vi "CONTROL TARGETING.vi"(8 "error in (no error)":errorcluster, 11 "control\ncluster":T1) -> (0 "error out":errorcluster, 3 "control\ncluster out":T1)   [LabVIEW 2023]
uses:
  ctrl defs/ctrl controllers.ctl
  Global odometry.vi
panel:
  in  "notes":string="ffsdfsdfsdf sdf sfsdf sdfsd sfds f sf sd fdsf \ndfdsf dsf sd fsd fsd\nsf sd fds fds fsdf ds fd"
  out "toggle\nTARGET?":bool
  in  "button for\nTARGET toggle":i32=6
  out "Buttons":bool[](array[boolean])
  out "POVs":i16[](array[numeric])
  out "Axes":dbl[](array[numeric])
  in  "axis scale":dbl=0.7 format="%#_13g"
  in  "axis dead band":dbl=0.025 format="%#_13g"
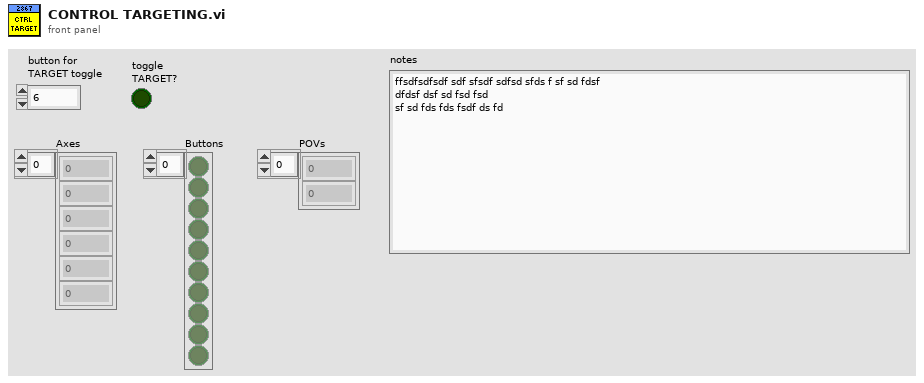
[diagram p1: front panel]
types:
  T1 = typedef "ctrl controllers.ctl" = cluster{"Axes":dbl[], "Buttons":bool[], "POVs":i16[]}
  T2 = typedef "ctrl LimeLight target.ctl" = cluster{"offsetAngle H":dbl, "offsetAngle V":dbl, "area":dbl, "skew":dbl, "driver assist":bool}
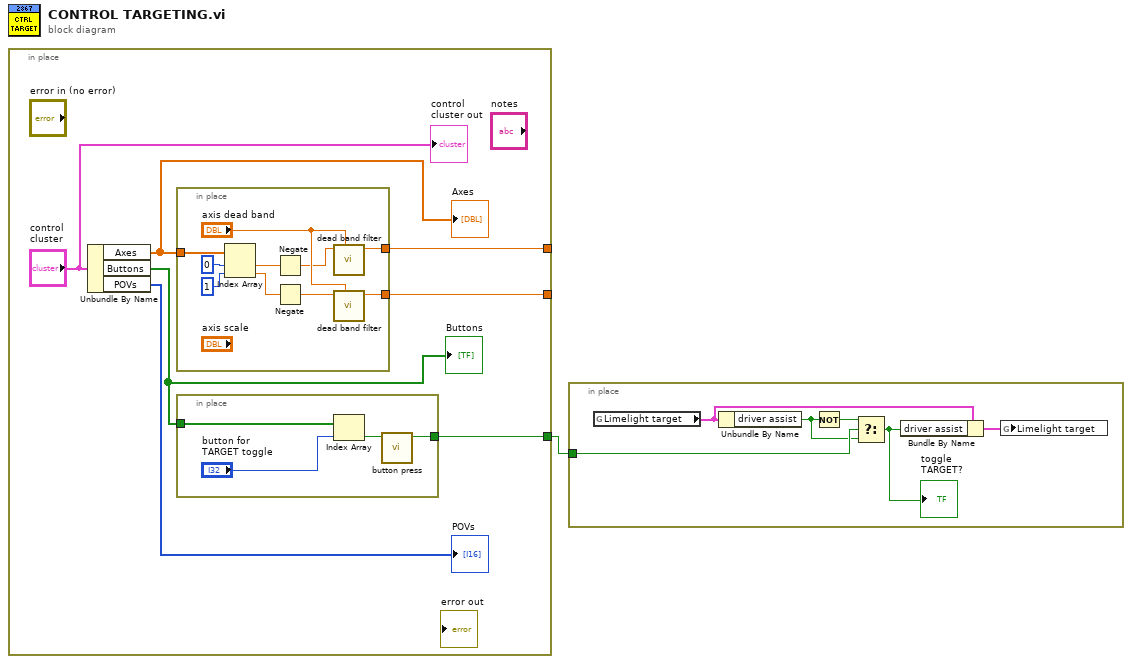
[diagram p0: block diagram]
diagram:
  n1 = in-place {
    in-place-border: [w8] -> _
    in-place-border: [w7] -> _
    in-place-border: [w2] -> w1
    n2 = Unbundle By Name("control\ncluster") -> ("Axes"=w5:dbl[], "Buttons"=w3:bool[], "POVs"=→"POVs":i16[])
    "Axes" <- w5
    "Buttons" <- w3
    n3 = in-place {
      in-place-border: [w15] -> w8
      in-place-border: [w14] -> w7
      in-place-border: w5 -> [w13]
      n4 = Index Array(array=w13, index #1=0 ("index"), index #2=1 ("index")) -> (element #1=w19:dbl, element #2=w18:dbl)
      n5 = Negate(x=w19) -> (-x=w17:dbl)
      n6 = Negate(x=w18) -> (-x=w16:dbl)
      n7 = call "dead band filter.vi"("deadband"="axis dead band", "input"=w17) -> ("output"=w15:dbl)  [unwired: 9 in]
      n8 = call "dead band filter.vi"("deadband"="axis dead band", "input"=w16) -> ("output"=w14:dbl)  [unwired: 9 in]
    }
    n9 = in-place {
      in-place-border: w3 -> [w12]
      in-place-border: [w9] -> w2
      n10 = Index Array(array=w12, index="button for\nTARGET toggle") -> (element=w11:bool)
      n11 = call "button press.vi"("button IN"=w11) -> ("Button Pressed?"=w9:bool)  [unwired: 10 in]
    }
    "control\ncluster out" <- "control\ncluster"
  }
  n12 = in-place {
    in-place-border: w1 -> [w27]
    n13 = global read "Global odometry.vi" "Limelight target"() -> (w26:T2)
    n14 = Unbundle By Name(w26) -> ("driver assist"=w25:bool)
    n15 = Not(x=w25) -> (.not. x?=w24:bool)
    n16 = Select(t=w24, s=w27, f=w25) -> (s? t:f=w23:bool)
    "toggle\nTARGET?" <- w23
    n17 = Bundle By Name(cluster=w26, "driver assist"=w23) -> (w28:T2)
    n18 = global write "Global odometry.vi" "Limelight target"(w28) -> ()
  }
